vi "recipeScript createPyUpperCode.vi"(7 "filePath":path, 8 "error in (no error)":errorcluster, 10 "instrTable":string[][](array[string]), 11 "userTable":string[][](array[string])) -> (0 "error out":errorcluster, 3 "concatenated string":string)   [LabVIEW 2018]
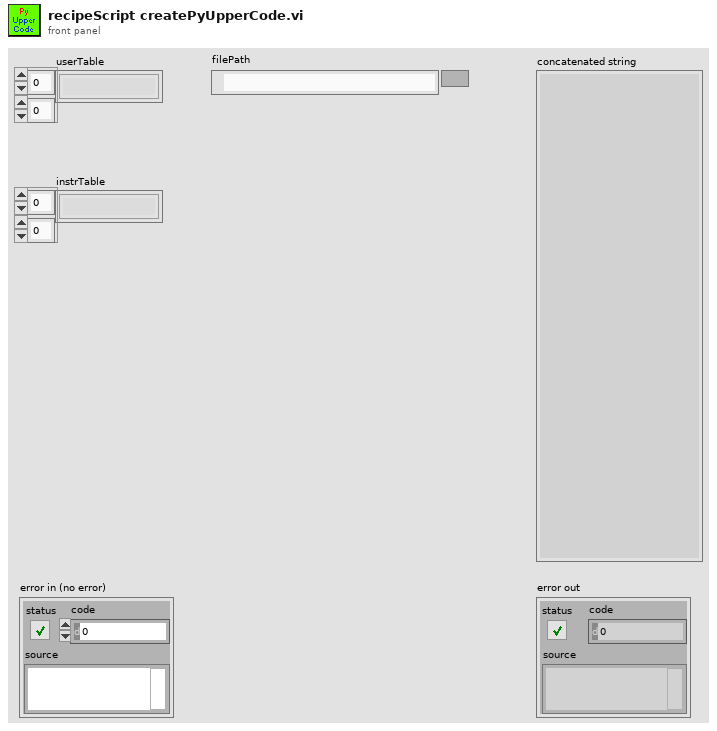
[diagram p1: front panel]
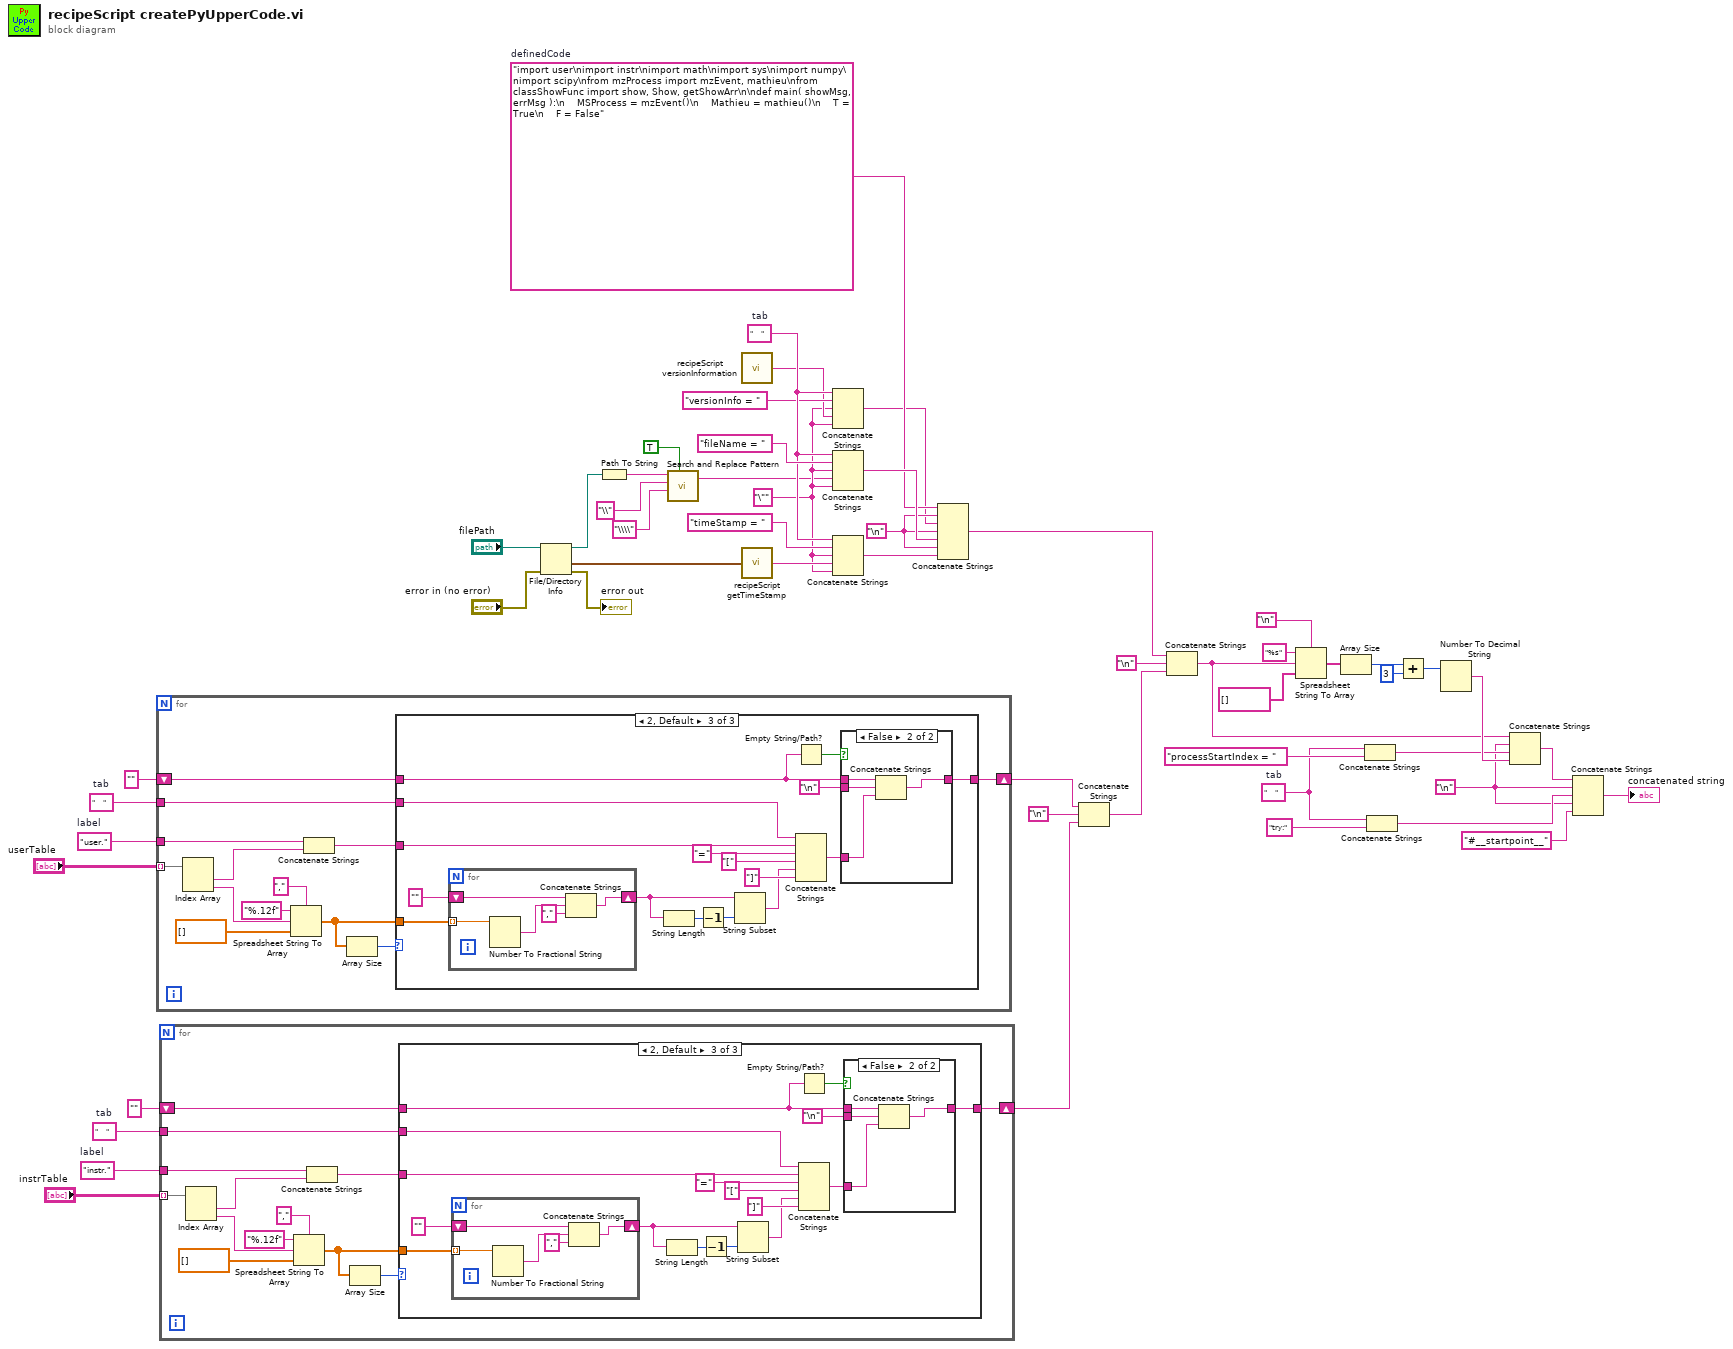
[diagram p0: block diagram]
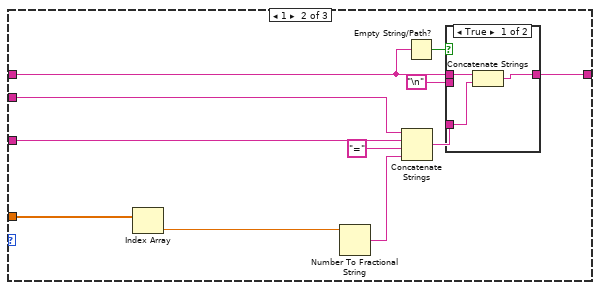
[diagram p3: hidden frame]
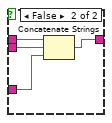
[diagram p4: hidden frame]
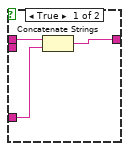
[diagram p5: hidden frame]
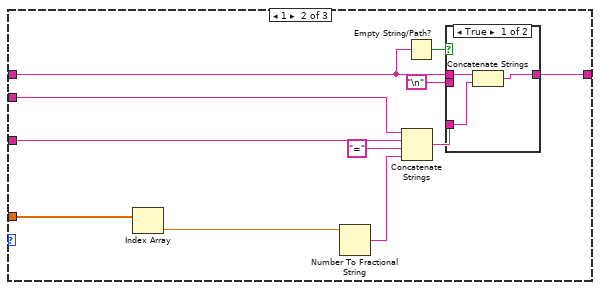
[diagram p7: hidden frame]
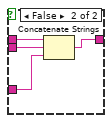
[diagram p8: hidden frame]
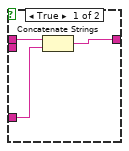
[diagram p9: hidden frame]
diagram:
  w11 = "user."  # label
  w12 = "    "  # tab
  w26 = "instr."  # label
  w28 = "    "  # tab
  w17 = "\""
  w15 = "\n"
  w20 = "    "  # tab
  w25 = "    "  # tab
  w16 = "import user\nimport instr\nimport math\nimport sys\nimport numpy\nimport scipy\nfrom mzProcess import mzEvent, mathieu\nfrom classShowFunc import show, Show, getShowArr\n\ndef main( showMsg, errMsg ):\n    MSProcess = mzEvent()\n    Mathieu = mathieu()\n    T = True\n    F = False"  # definedCode
  w24 = "\n"
  n1 = for {
    tunnel: "userTable" -> [w67] mode=indexing
    shift-right: [w59] -> w10
    shift-left: "" -> [w61]
    tunnel: w12 -> [w58]
    tunnel: w11 -> [w57]
    n2 = Index Array(array=w67) -> (element #1=w56:string, element #2=w66:string)  [unwired: 2 in]
    n3 = Spreadsheet String To Array(delimiter (Tab)=",", format string="%.12f", spreadsheet string=w66, array type (2D Dbl)=ext[] []) -> (array=w60:ext[])
    n4 = Concatenate Strings(w57, w56) -> (w55:string)
    n5 = Array Size(array=w60) -> (size(s)=w62:i32)
    n6 = case shown="2, Default" w62 {
      tunnel: w55 -> [_ w79 w102]
      tunnel: w61 -> [w68 w75 w99]
      tunnel: w60 -> [_ w77 w95]
      tunnel: [w68 w72 w96] -> w59
      tunnel: w58 -> [_ w69 w87]
      frame 0 {
      }
      frame 1 {
        n7 = Index Array(array=w77) -> (element=w76:ext)  [unwired: 1 in]
        n8 = Number To Fractional String(number=w76) -> (F-format string=w70:string)  [unwired: 3 in]
        n9 = Concatenate Strings(w69, w79, "=" ("string"), w70) -> (w74:string)
        n10 = Empty String/Path?(string/path=w75) -> (empty?=w73:bool)
        n11 = case shown="True" w73 {
          tunnel: "\n" -> [_ w84]
          tunnel: w75 -> [w82 w86]
          tunnel: w74 -> [w81 w83]
          tunnel: [w80 w85] -> w72
          frame True {
            n12 = Concatenate Strings(w82, w81) -> (w80:string)
          }
          frame False {
            n13 = Concatenate Strings(w86, w84, w83) -> (w85:string)
          }
        }
      }
      frame 2, Default {
        n14 = for {
          tunnel: w95 -> [w107] mode=indexing
          shift-right: [w104] -> w91
          shift-left: "" -> [w106]
          n15 = Number To Fractional String(number=w107) -> (F-format string=w105:string)  [unwired: 3 in]
          n16 = Concatenate Strings(w106, w105, "," ("string")) -> (w104:string)
        }
        n17 = String Length(string=w91) -> (length=w89:i32)
        n18 = Decrement(x=w89) -> (x-1=w88:i32)
        n19 = String Subset(string=w91, length (rest)=w88) -> (substring=w90:string)  [unwired: 1 in]
        n20 = Empty String/Path?(string/path=w99) -> (empty?=w97:bool)
        n21 = Concatenate Strings(w87, w102, "=" ("string"), "[" ("string"), w90, "]" ("string")) -> (w98:string)
        n22 = case shown="False" w97 {
          tunnel: "\n" -> [_ w112]
          tunnel: w99 -> [w110 w114]
          tunnel: w98 -> [w109 w111]
          tunnel: [w108 w113] -> w96
          frame True {
            n23 = Concatenate Strings(w110, w109) -> (w108:string)
          }
          frame False {
            n24 = Concatenate Strings(w114, w112, w111) -> (w113:string)
          }
        }
      }
    }
  }
  n25 = for {
    tunnel: "instrTable" -> [w127] mode=indexing
    shift-right: [w119] -> w8
    shift-left: "" -> [w121]
    tunnel: w28 -> [w118]
    tunnel: w26 -> [w117]
    n26 = Index Array(array=w127) -> (element #1=w116:string, element #2=w126:string)  [unwired: 2 in]
    n27 = Spreadsheet String To Array(delimiter (Tab)=",", format string="%.12f", spreadsheet string=w126, array type (2D Dbl)=ext[] []) -> (array=w120:ext[])
    n28 = Concatenate Strings(w117, w116) -> (w115:string)
    n29 = Array Size(array=w120) -> (size(s)=w122:i32)
    n30 = case shown="2, Default" w122 {
      tunnel: w115 -> [_ w139 w162]
      tunnel: w121 -> [w128 w135 w159]
      tunnel: w120 -> [_ w137 w155]
      tunnel: [w128 w132 w156] -> w119
      tunnel: w118 -> [_ w129 w147]
      frame 0 {
      }
      frame 1 {
        n31 = Index Array(array=w137) -> (element=w136:ext)  [unwired: 1 in]
        n32 = Number To Fractional String(number=w136) -> (F-format string=w130:string)  [unwired: 3 in]
        n33 = Concatenate Strings(w129, w139, "=" ("string"), w130) -> (w134:string)
        n34 = Empty String/Path?(string/path=w135) -> (empty?=w133:bool)
        n35 = case shown="True" w133 {
          tunnel: "\n" -> [_ w144]
          tunnel: w135 -> [w142 w146]
          tunnel: w134 -> [w141 w143]
          tunnel: [w140 w145] -> w132
          frame True {
            n36 = Concatenate Strings(w142, w141) -> (w140:string)
          }
          frame False {
            n37 = Concatenate Strings(w146, w144, w143) -> (w145:string)
          }
        }
      }
      frame 2, Default {
        n38 = for {
          tunnel: w155 -> [w167] mode=indexing
          shift-right: [w164] -> w151
          shift-left: "" -> [w166]
          n39 = Number To Fractional String(number=w167) -> (F-format string=w165:string)  [unwired: 3 in]
          n40 = Concatenate Strings(w166, w165, "," ("string")) -> (w164:string)
        }
        n41 = String Length(string=w151) -> (length=w149:i32)
        n42 = Decrement(x=w149) -> (x-1=w148:i32)
        n43 = String Subset(string=w151, length (rest)=w148) -> (substring=w150:string)  [unwired: 1 in]
        n44 = Empty String/Path?(string/path=w159) -> (empty?=w157:bool)
        n45 = Concatenate Strings(w147, w162, "=" ("string"), "[" ("string"), w150, "]" ("string")) -> (w158:string)
        n46 = case shown="False" w157 {
          tunnel: "\n" -> [_ w172]
          tunnel: w159 -> [w170 w174]
          tunnel: w158 -> [w169 w171]
          tunnel: [w168 w173] -> w156
          frame True {
            n47 = Concatenate Strings(w170, w169) -> (w168:string)
          }
          frame False {
            n48 = Concatenate Strings(w174, w172, w171) -> (w173:string)
          }
        }
      }
    }
  }
  n49 = File/Directory Info(path="filePath", error in="error in (no error)") -> (path out=w37:path, last mod=w22:timestamp, error out=→"error out":errorcluster)  [unwired: 4 out]
  n50 = Path To String(path=w37) -> (string=w1:string)
  n51 = call <vilib>:"Search and Replace Pattern.vi"("string"=w1, "regular expression (\"\")"="\\" ("regular expression (\"\")"), "replace string (\"\")"="\\\\" ("replace string (\"\")"), "replace all? (F)"=TRUE) -> ("result string"=w2:string)  [unwired: 1 in, 1 out]
  n52 = call "recipeScript versionInformation.vi"() -> ("verInfo"=w18:string)
  n53 = call "recipeScript getTimeStamp.vi"("timeFormat"=w22) -> ("timeStamp"=w21:string)
  n54 = Concatenate Strings(w20, "versionInfo = ", w17, w18, w17) -> (w14:string)
  n55 = Concatenate Strings(w20, "fileName = ", w17, w2, w17) -> (w32:string)
  n56 = Concatenate Strings(w20, "timeStamp = ", w17, w21, w17) -> (w31:string)
  n57 = Concatenate Strings(w16, w15, w14, w15, w32, w15, w31) -> (w30:string)
  n58 = Concatenate Strings(w10, "\n", w8) -> (w7:string)
  n59 = Concatenate Strings(w30, "\n", w7) -> (w46:string)
  n60 = Spreadsheet String To Array(delimiter (Tab)="\n", format string="%s", spreadsheet string=w46, array type (2D Dbl)=string[] []) -> (array=w51:string[])
  n61 = Array Size(array=w51) -> (size(s)=w41:i32)
  n62 = Concatenate Strings(w25, "processStartIndex = " ("string")) -> (w44:string)
  n63 = Concatenate Strings(w25, "try:" ("string")) -> (w42:string)
  n64 = Add(x=w41, y=3) -> (x+y=w39:i32)
  n65 = Number To Decimal String(number=w39) -> (decimal integer string=w50:string)  [unwired: 1 in]
  n66 = Concatenate Strings(w46, w24, w44, w50) -> (w49:string)
  n67 = Concatenate Strings(w49, w24, w42, w24, "#__startpoint__" ("string")) -> (→"concatenated string":string)
